vi "booleanRohit.vi"() -> ()   [LabVIEW 2009]
panel:
  in  "Enum":enum16{"and", "or", "nor", "nand"}(ring)
  out "Boolean 3":bool
  in  "Boolean 2":bool
  in  "Boolean":bool
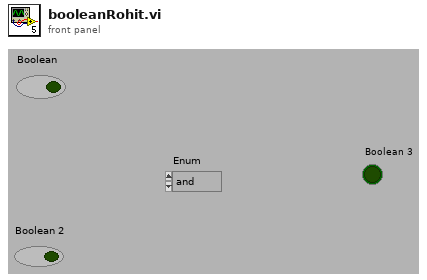
[diagram p1: front panel]
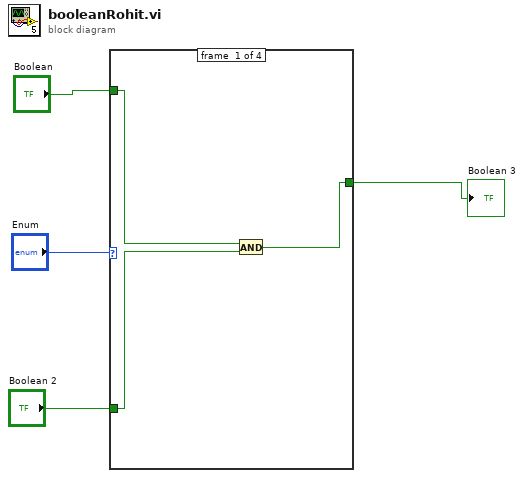
[diagram p0: block diagram]
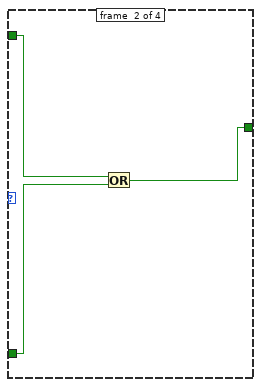
[diagram p2: hidden frame]
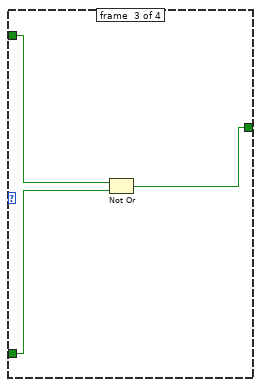
[diagram p3: hidden frame]
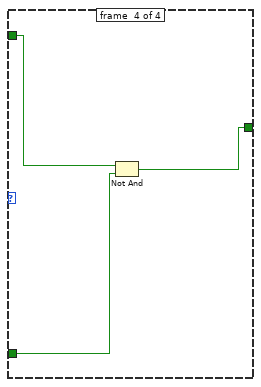
[diagram p4: hidden frame]
diagram:
  n1 = case shown="\"or\"" "Enum" {
    tunnel: "Boolean" -> [w7 w10 w13 w16]
    tunnel: "Boolean 2" -> [w6 w9 w12 w15]
    tunnel: [w5 w8 w11 w14] -> w2
    frame #0 {
      n2 = And(x=w7, y=w6) -> (x .and. y?=w5:bool)
    }
    frame #1 {
      n3 = Or(x=w10, y=w9) -> (x .or. y?=w8:bool)
    }
    frame #2 {
      n4 = Not Or(1:w12, 2:w13) -> (0:w11:bool)
    }
    frame #3 {
      n5 = Not And(1:w15, 2:w16) -> (0:w14:bool)
    }
  }
  "Boolean 3" <- w2
